vi "WFGenA04FM.vi"(1 "Param 0: Start Hz":dbl=20.0, 2 "Param 1: End Hz":dbl=200.0, 3 "Param 2: Inactive":dbl, 4 "Param 3: Inactive":dbl, 5 "error in (no error)":errorcluster, 8 "WFParameters":T2={"Fs (Hz)"=100000.0, "Amp (V)"=5.0, "Ramp (s)"=0.005, "Dur (s)"=0.25} {"Dur (s)" min=0.0 format="%#_4g"; "Ramp (s)" min=0.0; "Fs (Hz)" min=0.0}, 10 "WFRepetitions":T1={"Del (s)"=0.0, "Int (s)"=0.0, "N"=1} {"Int (s)" min=0.0 format="%#_4g"; "Del (s)" min=0.0 format="%#_4f"}) -> (14 "Waveform Out":waveform(dbl)={"t0"=timestamp(0 s since 1904-01-01), "dt"=1e-05, "Y"=array[25000 elements]}, 19 "error out":errorcluster)   [LabVIEW 2013]
uses:
  WFParameters.ctl
  WFRepetitions.ctl
  util/impl/WFComposeA.vi
panel:
  out "Waveform Graph":waveform(dbl)(graph)={"t0"=timestamp(0 s since 1904-01-01), "dt"=1e-05, "Y"=array[25000 elements]}
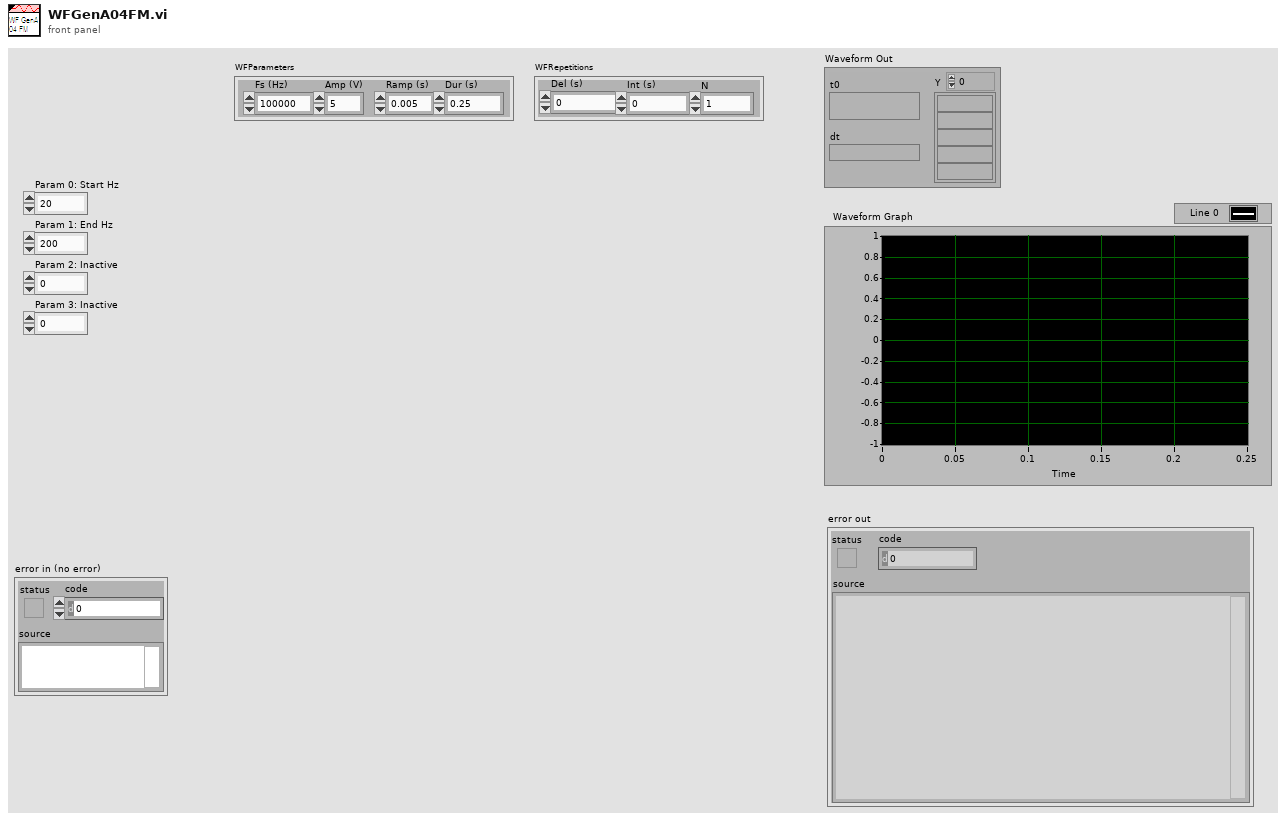
[diagram p1: front panel]
types:
  T1 = typedef "WFRepetitions.ctl" = cluster{"Del (s)":dbl, "Int (s)":dbl, "N":i32}
  T2 = typedef "WFParameters.ctl" = cluster{"Fs (Hz)":dbl, "Amp (V)":dbl, "Ramp (s)":dbl, "Dur (s)":dbl}
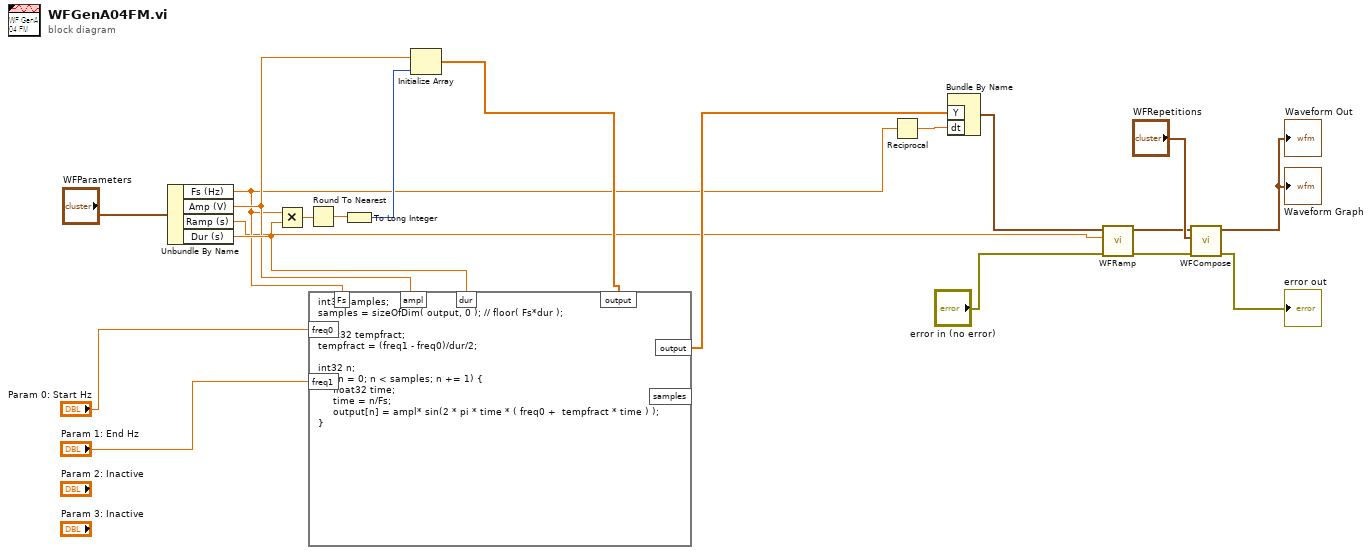
[diagram p0: block diagram]
diagram:
  n1 = Unbundle By Name("WFParameters") -> ("Fs (Hz)"=w8:dbl, "Amp (V)"=w9:dbl, "Ramp (s)"=w2:dbl, "Dur (s)"=w10:dbl)
  n2 = Multiply(x=w8, y=w10) -> (x*y=w15:dbl)
  n3 = Round To Nearest(number=w15) -> (nearest integer value=w14:dbl)
  n4 = To Long Integer(number=w14) -> (32bit integer=w17:i32)
  n5 = Initialize Array(w9, w17) -> (w13:dbl[])
  n6 = formula code="int32 samples;\nsamples = sizeOfDim( output, 0 ); // floor( Fs*dur );\n\nfloat32 tempfract;\ntempfract = (freq1 - freq0)/dur/2;\n\nint32 n;\nfor( n = 0; n < samples; n += 1) {\n     float32 time;\n     time = n/Fs;\n     output[n] = ampl* sin(2 * pi * time * ( freq0 +  tempfract * time ) );\n}"("dur"=w10, "freq0"="Param 0: Start Hz", "freq1"="Param 1: End Hz", "ampl"=w9, "Fs"=w8, "output"=w13) -> ("output"=w12:dbl[])  [unwired: 1 out]
  n7 = Reciprocal(x=w8) -> (1/x=w11:dbl)
  n8 = Bundle By Name("Y"=w12, "dt"=w11) -> (w3:waveform(dbl))  [unwired: 1 in]
  n9 = call "WFRamp.vi"("error in (no error)"="error in (no error)", "Ramp Length (s)"=w2, "Waveform In"=w3) -> ("error out"=w4:errorcluster, "Waveform Out"=w5:waveform(dbl))  [unwired: 7 in]
  n10 = call-poly "WFCompose.vi"("error in (no error)"=w4, "WFRepetitions"="WFRepetitions", "Waveform In"=w5) -> ("error out"=→"error out":errorcluster, "Analog Waveform Out"=→"Waveform Graph" →"Waveform Out":waveform(dbl))  [unwired: 7 in]
